vi "John's Video Viewer Find Timeout.vi"(1 "Status":T1) -> (0 "Timeout":i32)   [LabVIEW 2018]
uses:
  John's Video Viewer Status STYP.ctl
  Classes/Video File/Video File.lvclass
  Classes/Video Frame/Video Frame.lvclass
  Classes/Roughness Averager/Roughness Averager.lvclass
  Classes/Pointcloud/Pointcloud.lvclass
  <vilib>/vision/Image Controls.llb/IMAQ Image.ctl
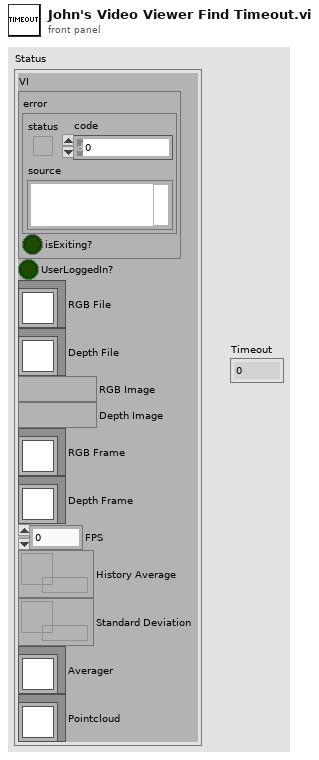
[diagram p1: front panel]
types:
  T1 = typedef "John's Video Viewer Status STYP.ctl" = cluster{"VI":cluster{"error":errorcluster, "isExiting?":bool}, "UserLoggedIn?":bool, "RGB File":refnum<class "Video File.lvclass">, "Depth File":refnum<class "Video File.lvclass">, "RGB Image":T2, "Depth Image":T2, "RGB Frame":refnum<class "Video Frame.lvclass">, "Depth Frame":refnum<class "Video Frame.lvclass">, "FPS":i32, "History Average":refnum<queue>, "Standard Deviation":refnum<queue>, "Averager":refnum<class "Roughness Averager.lvclass">, "Pointcloud":refnum<class "Pointcloud.lvclass">}
  T2 = typedef "IMAQ Image.ctl" = refnum<image>
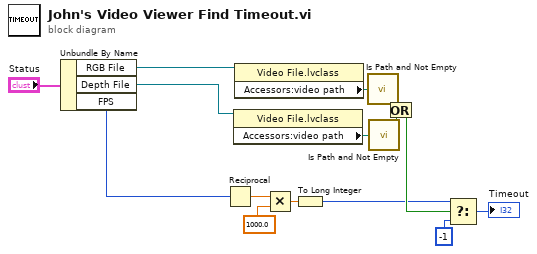
[diagram p0: block diagram]
diagram:
  n1 = Unbundle By Name("Status") -> ("RGB File"=w14:refnum<class "Video File.lvclass">, "Depth File"=w13:refnum<class "Video File.lvclass">, "FPS"=w7:i32)
  n2 = Reciprocal(x=w7) -> (1/x=w6:dbl)
  n3 = property class="Video File.lvclass"(reference=w13) -> ("Accessors:video path"=w11:path)  [unwired: 1 in, 2 out]
  n4 = property class="Video File.lvclass"(reference=w14) -> ("Accessors:video path"=w12:path)  [unwired: 1 in, 2 out]
  n5 = Multiply(x=w6, y=1000.0) -> (x*y=w4:dbl)
  n6 = To Long Integer(number=w4) -> (32bit integer=w2:i32)
  n7 = call <vilib>:"Is Path and Not Empty.vi"("path"=w12) -> ("Is Path and Not Empty?"=w10:bool)  [unwired: 4 in]
  n8 = call <vilib>:"Is Path and Not Empty.vi"("path"=w11) -> ("Is Path and Not Empty?"=w9:bool)  [unwired: 4 in]
  n9 = Or(x=w10, y=w9) -> (x .or. y?=w8:bool)
  n10 = Select(t=w2, s=w8, f=-1 ("t")) -> (s? t:f=→"Timeout":i32)
